vi "Write Boolean.vi"(8 "error in (no error)":errorcluster, 10 "Numeric":dbl, 11 "ExampleClass2 in":refnum<class "ExampleClass2.lvclass">) -> (0 "error out":errorcluster, 3 "ExampleClass2 out":refnum<class "ExampleClass2.lvclass">)   [LabVIEW 2014, in "ExampleClass2.lvclass"]
uses:
  ExampleClass2.lvclass
  ExampleClass2.lvclass/ExampleClass2.ctl
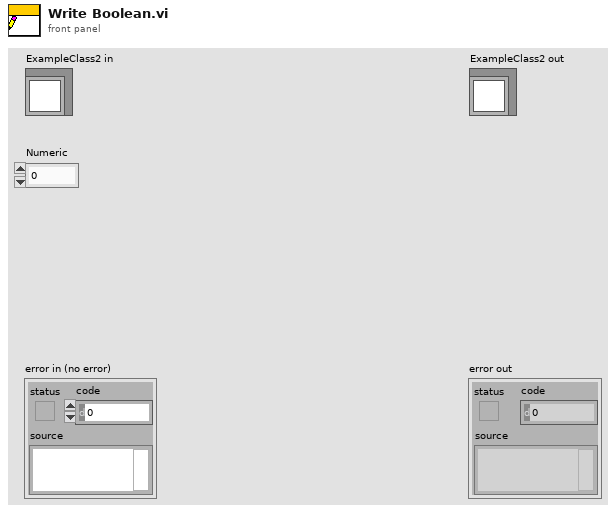
[diagram p1: front panel]
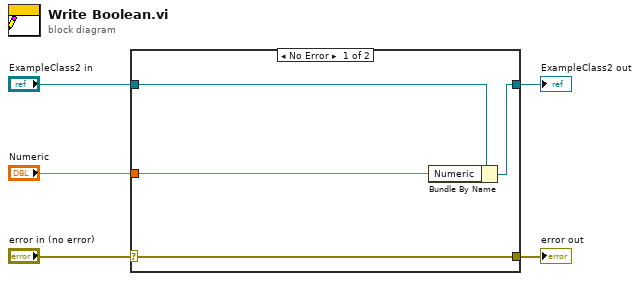
[diagram p0: block diagram]
diagram:
  n1 = case shown="No Error" "error in (no error)" {
    selector: "error in (no error)" -> [w9 w10]
    tunnel: [w9 w10] -> w4
    tunnel: [w7 w11] -> w2
    tunnel: "ExampleClass2 in" -> [w8 w11]
    tunnel: "Numeric" -> [w6 _]
    frame No Error {
      n2 = Bundle By Name(cluster=w8, "Numeric"=w6) -> (w7:refnum<class "ExampleClass2.lvclass">)
    }
    frame Error {
    }
  }
  "error out" <- w4
  "ExampleClass2 out" <- w2
